vi "Command.vi"(8 "error in (no error)":errorcluster, 10 "command":string, 11 "MKS MW in":refnum<class "PL MKS MW.lvclass">) -> (0 "error out":errorcluster, 2 "response data":string, 3 "MKS MW out":refnum<class "PL MKS MW.lvclass">)   [LabVIEW 2015, in "PL MKS MW.lvclass"]
doc: "Sends <b>command</b> to device and returns <b>response data</b>."
uses:
  PL MKS MW.lvclass
  PL MKS MW.lvclass/PL MKS MW.ctl
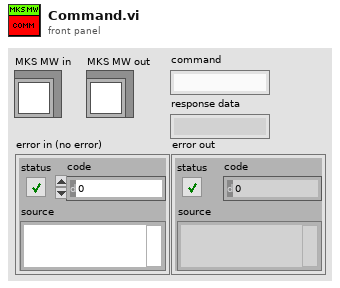
[diagram p1: front panel]
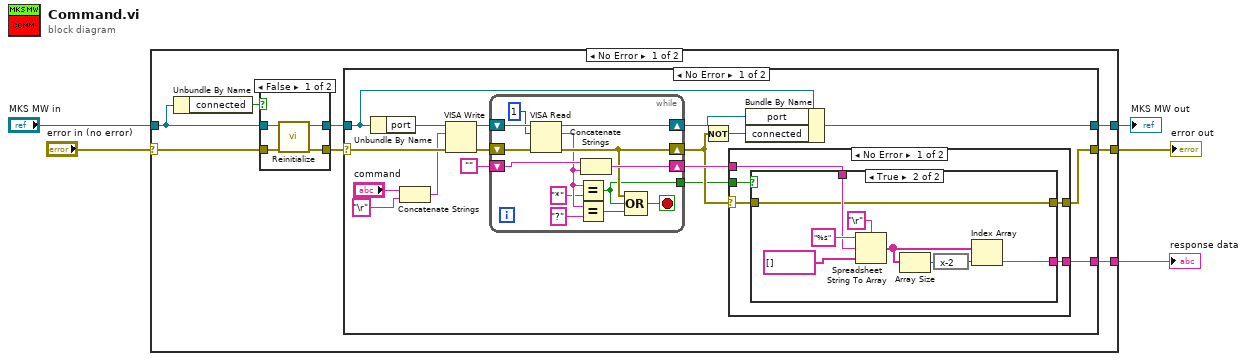
[diagram p0: block diagram]
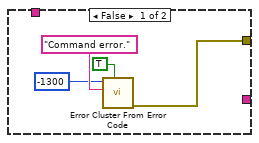
[diagram p2: hidden frame]
diagram:
  n1 = case shown="No Error" "error in (no error)" {
    selector: "error in (no error)" -> [w11 w72]
    tunnel: "MKS MW in" -> [w12 w71]
    tunnel: [w8 w72] -> w2
    tunnel: [w7 w71] -> w3
    tunnel: [w6 _] -> w1
    frame No Error {
      n2 = Unbundle By Name(w12) -> ("connected"=w13:bool)
      n3 = case shown="False" w13 {
        tunnel: w12 -> [w68 w70]
        tunnel: w11 -> [w67 w69]
        tunnel: [w66 w70] -> w9
        tunnel: [w65 w69] -> w10
        frame False {
          n4 = call "Reinitialize.vi"("error in (no error)"=w67, "MKS MW in"=w68) -> ("error out"=w65:errorcluster, "MKS MW out"=w66:refnum<class "PL MKS MW.lvclass">)  [unwired: 8 in]
        }
        frame True {
        }
      }
      n5 = case shown="No Error" w10 {
        selector: w10 -> [w27 w64]
        tunnel: w9 -> [w23 w63]
        tunnel: [w14 w64] -> w8
        tunnel: [w20 w63] -> w7
        tunnel: [w17 _] -> w6
        frame No Error {
          n6 = Unbundle By Name(w23) -> ("port"=w30:refnum<visa-resource-name>)
          n7 = Concatenate Strings("command", "\r" ("string")) -> (w24:string)
          n8 = VISA Write(VISA resource name=w30, write buffer=w24, error in (no error)=w27) -> (VISA resource name out=w29:refnum<visa-resource-name>, error out=w28:errorcluster)  [unwired: 1 out]
          n9 = while {
            shift-right: [w60] -> w22
            shift-left: w29 -> [w62]
            shift-right: [w56] -> w16
            shift-left: w28 -> [w61]
            shift-right: [w58] -> w18
            shift-left: "" -> [w57]
            tunnel: [w50] -> w15
            stop <- w55 stop-if-true
            n10 = VISA Read(VISA resource name=w62, byte count=u32 1, error in (no error)=w61) -> (VISA resource name out=w60:refnum<visa-resource-name>, read buffer=w53:string, error out=w56:errorcluster)  [unwired: 1 out]
            n11 = Equal?(x=w53, y="*") -> (x = y?=w50:bool)
            n12 = Equal?(x=w53, y="?") -> (x = y?=w54:bool)
            n13 = Concatenate Strings(w57, w53) -> (w58:string)
            n14 = Compound Arithmetic op=OR(w56, w50, w54) -> (w55:bool)
          }
          n15 = Not(x=w16) -> (.not. x?=w21:bool)
          n16 = case shown="No Error" w16 {
            selector: w16 -> [w32 w49]
            tunnel: w18 -> [w35 _]
            tunnel: [w34 _] -> w17
            tunnel: w15 -> [w33 _]
            tunnel: [w31 w49] -> w14
            frame No Error {
              n17 = case shown="True" w33 {
                tunnel: w35 -> [_ w43]
                tunnel: [_ w40] -> w34
                tunnel: w32 -> [_ w41]
                tunnel: [w36 w41] -> w31
                frame False {
                  n18 = call <vilib>:"Error Cluster From Error Code.vi"("show call chain? (False)"=TRUE, "error message (\"\")"="Command error." ("format string"), "error code (0)"=-1300) -> ("error out"=w36:errorcluster)  [unwired: 6 in]
                }
                frame True {
                  n19 = Spreadsheet String To Array(delimiter (Tab)="\r", format string="%s", spreadsheet string=w43, array type (2D Dbl)=string[] []) -> (array=w46:string[])
                  n20 = Array Size(array=w46) -> (size(s)=w45:i32)
                  n21 = expression code="x-2"(w45) -> (w44:i32)
                  n22 = Index Array(array=w46, index=w44) -> (element=w40:string)
                }
              }
            }
            frame Error {
            }
          }
          n23 = Bundle By Name(cluster=w23, "port"=w22, "connected"=w21) -> (w20:refnum<class "PL MKS MW.lvclass">)
        }
        frame Error {
        }
      }
    }
    frame Error {
    }
  }
  "MKS MW out" <- w3
  "response data" <- w1
  "error out" <- w2
